vi "cost.vi"(8 "error in (no error)":errorcluster, 11 "Decaf in":refnum<class "Decaf.lvclass">) -> (0 "error out":errorcluster, 2 "Cost":dbl, 3 "Decaf out":refnum<class "Decaf.lvclass">)   [LabVIEW 2013, in "Decaf.lvclass"]
uses:
  Decaf.lvclass
  Beverage/Beverage.lvclass
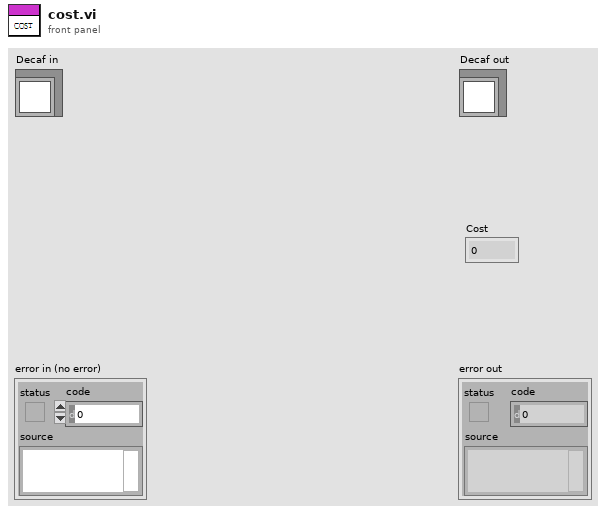
[diagram p1: front panel]
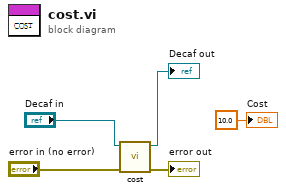
[diagram p0: block diagram]
diagram:
  n1 = call-parent "cost.vi"("error in (no error)"="error in (no error)", "Beverage in"="Decaf in") -> ("error out"=→"error out":errorcluster, "Beverage out"=→"Decaf out":refnum<class "Decaf.lvclass">)  [unwired: 7 in, 1 out]
  "Cost" <- 10.0 ("Cost")
